vi "Read2 Channels Metodo.vi"(6 "Measurement Type (0: Phase)":i32(ring) items=["Phase", "Delay", "DelayRR", "DelayRF", "DelayFR", "DelayFF"], 8 "error in (no error)":errorcluster, 9 "Channels":T1={"Data Tektronix"={"Channel 1 (1: Channel 1)"=1, "Channel 2 (2: Channel 2)"=2}, "Data Edu"={"Channels 2"=[], "Timeout (10000 ms)"=10000}} {"Data Edu"."Channels 2" items=["Channel 1"=0, "Channel 2"=1, "Channel 3"=2, "Channel 4"=3, "Waveform Memory 1"=5, "Waveform Memory 2"=6, "Serial Bus 1"=7, "Serial Bus 2"=8, "Digital Bus Low"=9, "Digital Bus High "=10, "Digital Bus 1"=11, "Digital Bus 2"=12, "External"=29, "Function 1"=32, "Function 2"=33, "Function 3"=34, "Function 4"=35, "Math 1"=36, "Math 2"=37, "Math 3"=38, "Math 4"=39, "FFT"=40, "Analog Bus"=41]; "Data Tektronix"."Channel 2 (2: Channel 2)" items=["Channel 1"=1, "Channel 2"=2, "Channel 3"=3, "Channel 4"=4]; "Data Tektronix"."Channel 1 (1: Channel 1)" items=["Channel 1"=1, "Channel 2"=2, "Channel 3"=3, "Channel 4"=4]}, 11 "Keysight in":refnum<class "Edu-1200.lvclass">) -> (0 "error out":errorcluster, 1 "Data Out":T2, 3 "Keysight out":refnum<class "Edu-1200.lvclass">)   [LabVIEW 2020, in "Edu-1200.lvclass"]
uses:
  Edu-1200.lvclass
  Edu-1200.lvclass/Edu-1200.ctl
  <instrlib>/Agilent 2000 3000 X-Series/Public/Data/Read Waveforms (Multiple).vi
  <instrlib>/Agilent 2000 3000 X-Series/Agilent 2000 3000 X-Series.lvlib
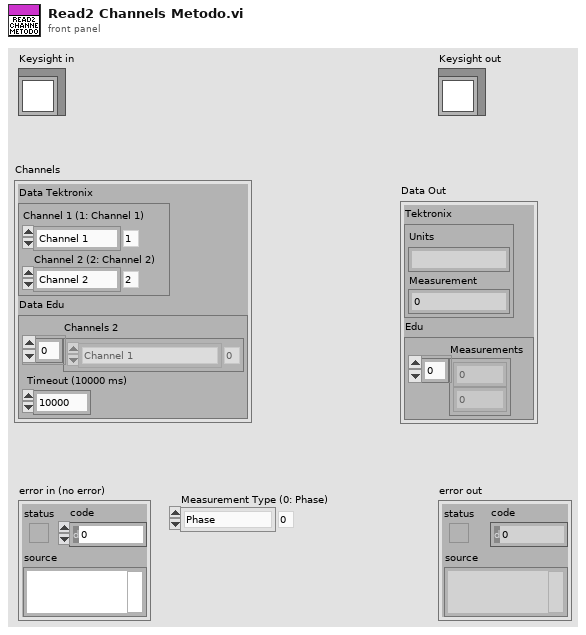
[diagram p1: front panel]
types:
  T1 = cluster{"Data Tektronix":cluster{"Channel 1 (1: Channel 1)":i32, "Channel 2 (2: Channel 2)":i32}, "Data Edu":cluster{"Channels 2":i32[], "Timeout (10000 ms)":u32}}
  T2 = cluster{"Tektronix":cluster{"Units":string, "Measurement":dbl}, "Edu":cluster{"Measurements":dbl[]}}
  T3 = cluster{"Tektronix":cluster{"Units":string, "Measurement":dbl}, "Keysight":cluster{"Measurements":dbl[]}}
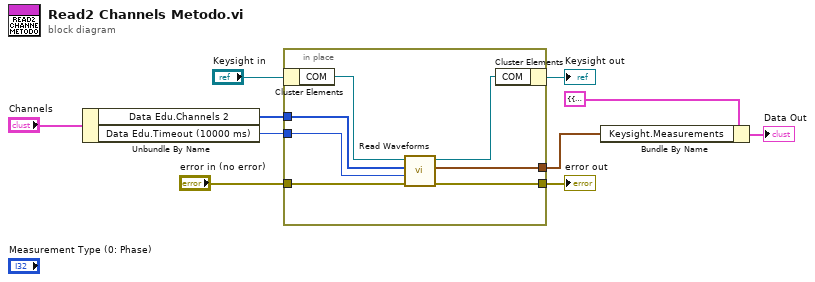
[diagram p0: block diagram]
diagram:
  n1 = Unbundle By Name("Channels") -> ("Data Edu.Channels 2"=w5:i32[], "Data Edu.Timeout (10000 ms)"=w4:u32)
  n2 = in-place {
    in-place-border: "error in (no error)" -> [w17]
    in-place-border: [w16] -> w7
    in-place-border: w5 -> [w12]
    in-place-border: w4 -> [w11]
    in-place-border: [w13] -> w1
    n3 = in-place-cluster #1("Keysight in") -> ("COM"=w15:refnum<visa-resource-name>)
    n4 = call-poly <instrlib>:"Read Waveforms.vi"("error in (no error)"=w17, "Timeout (10000 ms)"=w11, "Channels"=w12, "VISA resource name"=w15) -> ("error out"=w16:errorcluster, "Waveform Data"=w13:waveform(dbl)[], "VISA resource name out"=w14:refnum<visa-resource-name>)  [unwired: 5 in]
    n5 = in-place-cluster #1("COM"=w14) -> (→"Keysight out":refnum<class "Edu-1200.lvclass">)
  }
  "error out" <- w7
  n6 = Bundle By Name(cluster=T3 {"Tektronix"={"Units"="", "Measurement"=0.0}, "Keysight"={"Measurements"=[]}} ("Data Out"), "Keysight.Measurements"=w1) -> (→"Data Out":T3)
